vi "data parsing.vi"(11 "문자열":string) -> (0 "Right 3":T1, 1 "Right 2":T1, 2 "Right 1":T1, 3 "Left 3":T1, 4 "Left_Sum":u32[](array[numeric]), 5 "Left 2":T1, 6 "Right_Sum":u32[](array[numeric]), 7 "Left 1":T1, 8 "Time(s)":dbl[](array[numeric]))   [LabVIEW 2015]
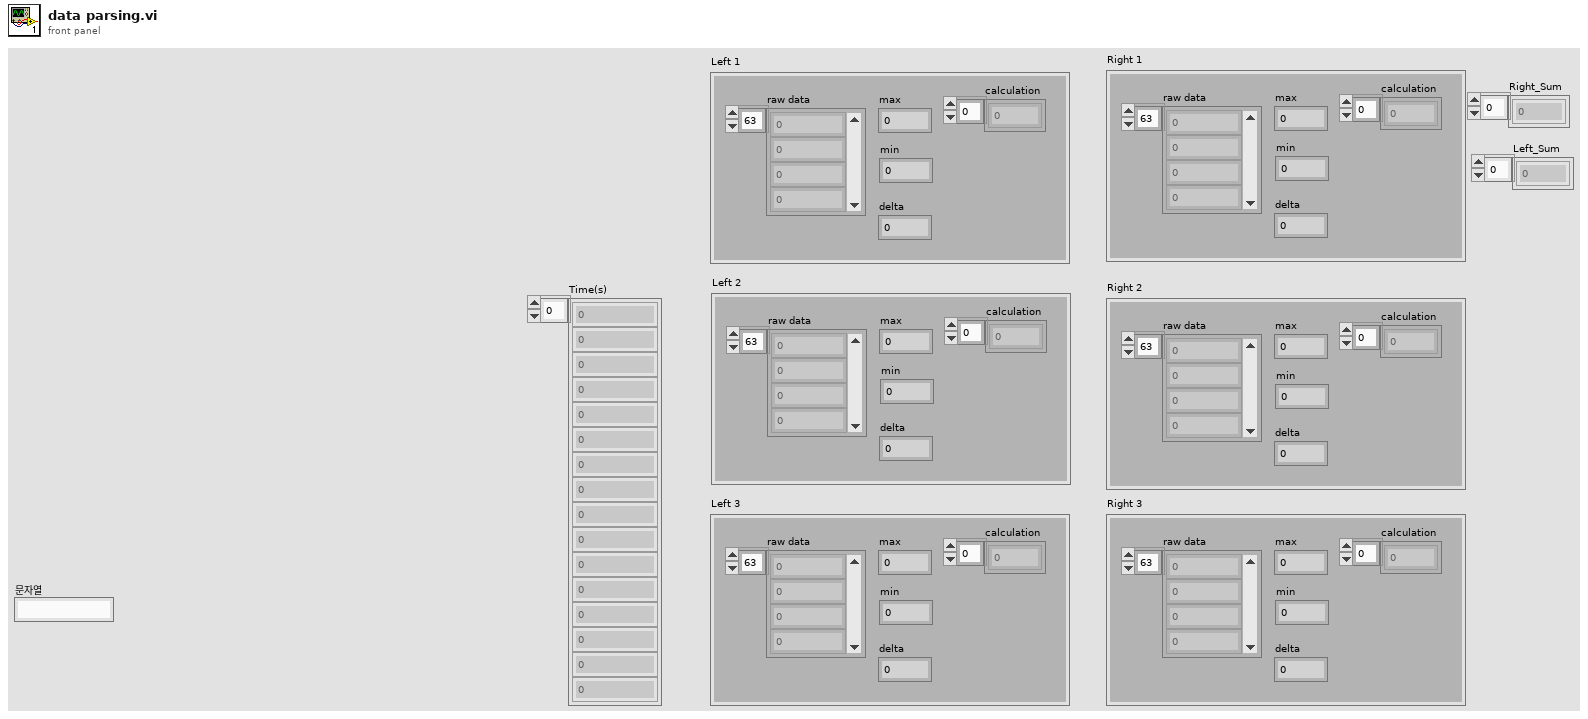
[diagram p1: front panel]
types:
  T1 = cluster{"raw data":u32[], "max":u32, "min":u32, "delta":u32, "calculation":u32[]}
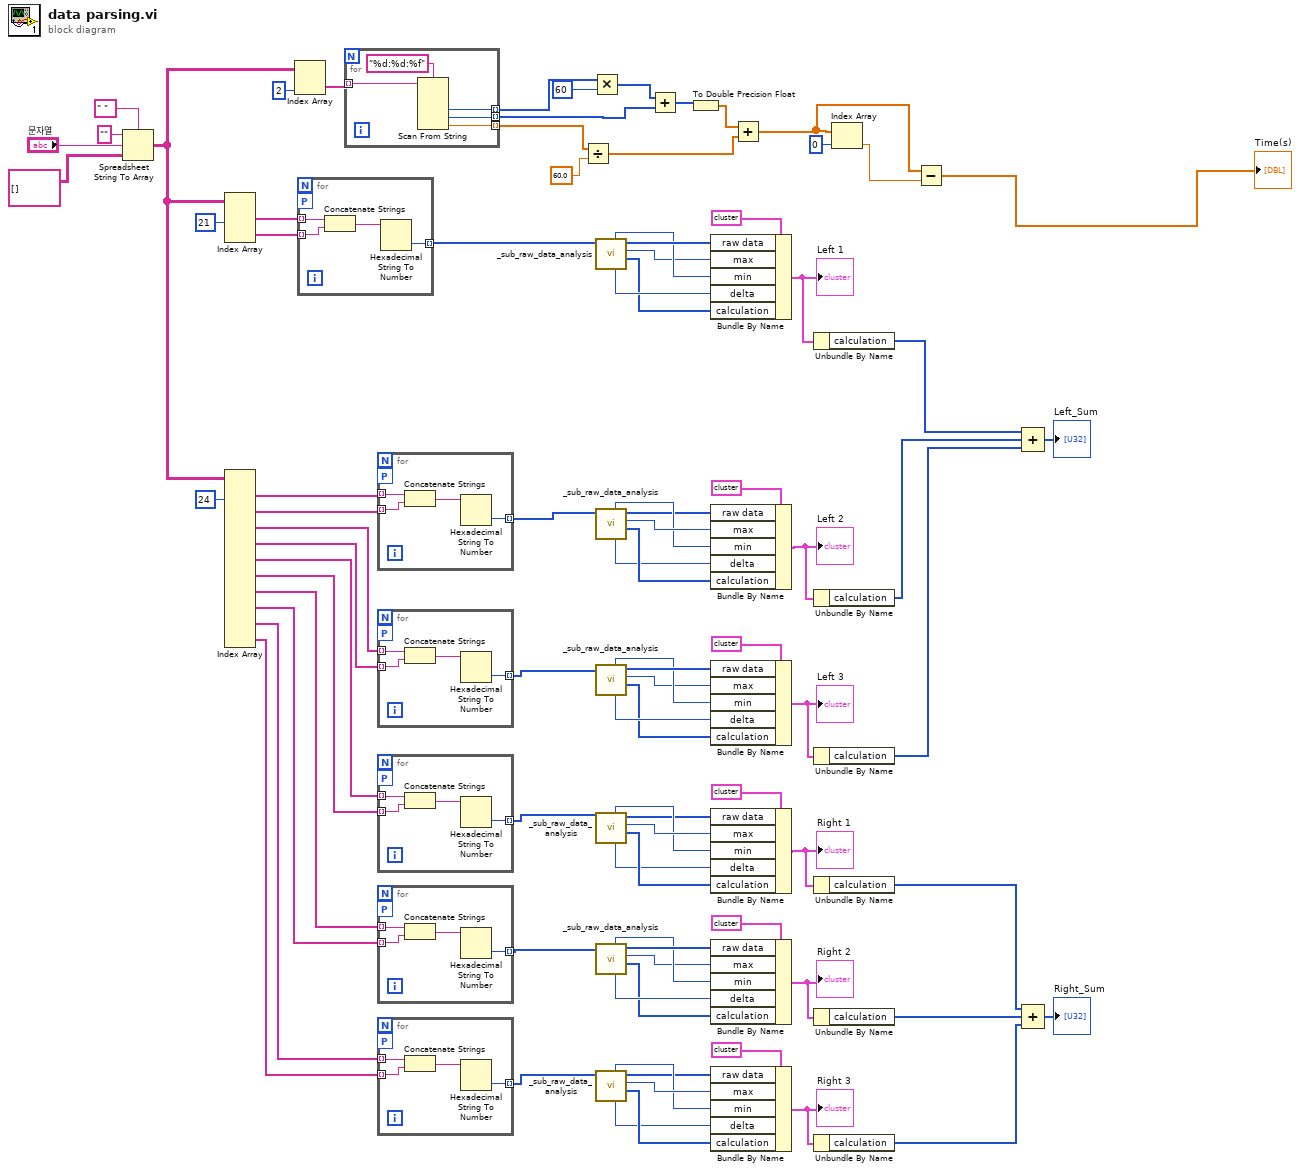
[diagram p0: block diagram]
diagram:
  n1 = Spreadsheet String To Array(delimiter (Tab)=" " ("구분 문자(탭)"), format string="", spreadsheet string="문자열", array type (2D Dbl)=string[][] []) -> (array=w72:string[][])
  n2 = Index Array(array=w72, index (col) #1=21 ("비활성화된 인덱스 (열)")) -> (element #1=w85:string[], element #2=w84:string[])  [unwired: 3 in]
  n3 = Index Array(array=w72, index (col) #1=24 ("비활성화된 인덱스 (열)")) -> (element #1=w82:string[], element #2=w81:string[], element #3=w80:string[], element #4=w79:string[], element #5=w78:string[], element #6=w77:string[], element #7=w76:string[], element #8=w75:string[], element #9=w74:string[], element #10=w73:string[])  [unwired: 19 in]
  n4 = Index Array(array=w72, index (col)=2 ("비활성화된 인덱스 (열)")) -> (element=w70:string[])  [unwired: 1 in]
  n5 = for {
    tunnel: w85 -> [w94] mode=indexing
    tunnel: w84 -> [w93] mode=indexing
    tunnel: [w91] -> w6 mode=indexing
    workers-P: _ -> [_]
    n6 = Concatenate Strings(w94, w93) -> (w92:string)
    n7 = Hexadecimal String To Number(string=w92) -> (number=w91:u32)  [unwired: 2 in, 1 out]
  }
  n8 = for {
    tunnel: w70 -> [w99] mode=indexing
    tunnel: [w97] -> w68 mode=indexing
    tunnel: [w96] -> w11 mode=indexing
    tunnel: [w95] -> w10 mode=indexing
    n9 = Scan From String(format string="%d:%d:%f" ("포맷 문자열"), input string=w99) -> (output 1=w97:i32, output 2=w96:i32, output 3=w95:dbl)  [unwired: 5 in, 3 out]
  }
  n10 = for {
    tunnel: w82 -> [w103] mode=indexing
    tunnel: w81 -> [w102] mode=indexing
    tunnel: [w100] -> w5 mode=indexing
    workers-P: _ -> [_]
    n11 = Concatenate Strings(w103, w102) -> (w101:string)
    n12 = Hexadecimal String To Number(string=w101) -> (number=w100:u32)  [unwired: 2 in, 1 out]
  }
  n13 = for {
    tunnel: w80 -> [w107] mode=indexing
    tunnel: w79 -> [w106] mode=indexing
    tunnel: [w104] -> w4 mode=indexing
    workers-P: _ -> [_]
    n14 = Concatenate Strings(w107, w106) -> (w105:string)
    n15 = Hexadecimal String To Number(string=w105) -> (number=w104:u32)  [unwired: 2 in, 1 out]
  }
  n16 = for {
    tunnel: w78 -> [w111] mode=indexing
    tunnel: w77 -> [w110] mode=indexing
    tunnel: [w108] -> w3 mode=indexing
    workers-P: _ -> [_]
    n17 = Concatenate Strings(w111, w110) -> (w109:string)
    n18 = Hexadecimal String To Number(string=w109) -> (number=w108:u32)  [unwired: 2 in, 1 out]
  }
  n19 = for {
    tunnel: w76 -> [w115] mode=indexing
    tunnel: w75 -> [w114] mode=indexing
    tunnel: [w112] -> w2 mode=indexing
    workers-P: _ -> [_]
    n20 = Concatenate Strings(w115, w114) -> (w113:string)
    n21 = Hexadecimal String To Number(string=w113) -> (number=w112:u32)  [unwired: 2 in, 1 out]
  }
  n22 = for {
    tunnel: w74 -> [w119] mode=indexing
    tunnel: w73 -> [w118] mode=indexing
    tunnel: [w116] -> w1 mode=indexing
    workers-P: _ -> [_]
    n23 = Concatenate Strings(w119, w118) -> (w117:string)
    n24 = Hexadecimal String To Number(string=w117) -> (number=w116:u32)  [unwired: 2 in, 1 out]
  }
  n25 = Divide(x=w10, y=60.0) -> (x/y=w8:dbl[])
  n26 = Multiply(x=w68, y=60) -> (x*y=w67:i32[])
  n27 = call "_sub_raw_data_analysis.vi"("raw data input"=w6) -> ("Raw-Del"=w57:u32[], "MAX"=w59:u32, "raw data output"=w61:u32[], "LWA_DEL"=w58:u32, "MIN"=w60:u32)  [unwired: 6 in]
  n28 = call "_sub_raw_data_analysis.vi"("raw data input"=w5) -> ("Raw-Del"=w56:u32[], "MAX"=w54:u32, "raw data output"=w52:u32[], "LWA_DEL"=w55:u32, "MIN"=w53:u32)  [unwired: 6 in]
  n29 = call "_sub_raw_data_analysis.vi"("raw data input"=w4) -> ("Raw-Del"=w45:u32[], "MAX"=w47:u32, "raw data output"=w49:u32[], "LWA_DEL"=w46:u32, "MIN"=w48:u32)  [unwired: 6 in]
  n30 = call "_sub_raw_data_analysis.vi"("raw data input"=w3) -> ("Raw-Del"=w44:u32[], "MAX"=w42:u32, "raw data output"=w40:u32[], "LWA_DEL"=w43:u32, "MIN"=w41:u32)  [unwired: 6 in]
  n31 = call "_sub_raw_data_analysis.vi"("raw data input"=w2) -> ("Raw-Del"=w33:u32[], "MAX"=w35:u32, "raw data output"=w37:u32[], "LWA_DEL"=w34:u32, "MIN"=w36:u32)  [unwired: 6 in]
  n32 = call "_sub_raw_data_analysis.vi"("raw data input"=w1) -> ("Raw-Del"=w32:u32[], "MAX"=w30:u32, "raw data output"=w28:u32[], "LWA_DEL"=w31:u32, "MIN"=w29:u32)  [unwired: 6 in]
  n33 = Add(x=w67, y=w11) -> (x+y=w65:i32[])
  n34 = To Double Precision Float(number=w65) -> (double precision float=w66:dbl[])
  n35 = Bundle By Name(cluster=T1 {"raw data"=array[319065 elements], "max"=0, "min"=0, "delta"=0, "calculation"=[]} ("LWA"), "raw data"=w61, "max"=w59, "min"=w60, "delta"=w58, "calculation"=w57) -> (w26:T1)
  "Left 1" <- w26
  n36 = Bundle By Name(cluster=T1 {"raw data"=array[319065 elements], "max"=0, "min"=0, "delta"=0, "calculation"=[]} ("LWA"), "raw data"=w52, "max"=w54, "min"=w53, "delta"=w55, "calculation"=w56) -> (w25:T1)
  "Left 2" <- w25
  n37 = Bundle By Name(cluster=T1 {"raw data"=array[319065 elements], "max"=0, "min"=0, "delta"=0, "calculation"=[]} ("LWA"), "raw data"=w49, "max"=w47, "min"=w48, "delta"=w46, "calculation"=w45) -> (w24:T1)
  "Left 3" <- w24
  n38 = Bundle By Name(cluster=T1 {"raw data"=array[319065 elements], "max"=0, "min"=0, "delta"=0, "calculation"=[]} ("LWA"), "raw data"=w40, "max"=w42, "min"=w41, "delta"=w43, "calculation"=w44) -> (w23:T1)
  "Right 1" <- w23
  n39 = Bundle By Name(cluster=T1 {"raw data"=array[319065 elements], "max"=0, "min"=0, "delta"=0, "calculation"=[]} ("LWA"), "raw data"=w37, "max"=w35, "min"=w36, "delta"=w34, "calculation"=w33) -> (w22:T1)
  "Right 2" <- w22
  n40 = Bundle By Name(cluster=T1 {"raw data"=array[319065 elements], "max"=0, "min"=0, "delta"=0, "calculation"=[]} ("LWA"), "raw data"=w28, "max"=w30, "min"=w29, "delta"=w31, "calculation"=w32) -> (w21:T1)
  "Right 3" <- w21
  n41 = Add(x=w66, y=w8) -> (x+y=w12:dbl[])
  n42 = Unbundle By Name(w26) -> ("calculation"=w20:u32[])
  n43 = Unbundle By Name(w25) -> ("calculation"=w18:u32[])
  n44 = Unbundle By Name(w24) -> ("calculation"=w19:u32[])
  n45 = Unbundle By Name(w23) -> ("calculation"=w16:u32[])
  n46 = Unbundle By Name(w22) -> ("calculation"=w17:u32[])
  n47 = Unbundle By Name(w21) -> ("calculation"=w15:u32[])
  n48 = Index Array(array=w12, index=0 ("인덱스")) -> (element=w63:dbl)
  n49 = Subtract(x=w12, y=w63) -> (x-y=→"Time(s)":dbl[])
  n50 = Compound Arithmetic op=ADD(w20, w18, w19) -> (→"Left_Sum":u32[])
  n51 = Compound Arithmetic op=ADD(w16, w17, w15) -> (→"Right_Sum":u32[])
